vi "Add Page Attachements.vi"(6 "Parallel?":bool, 7 "Conf Printer in":refnum<class "VIDoc Printer - Confluence.lvclass">, 8 "error in (no error)":errorcluster, 9 "Msg Chain in":string, 10 "Attachments":set{path}(c389), 11 "Page in":refnum<class "Page.lvclass">) -> (0 "error out":errorcluster, 3 "Page out":refnum<class "Page.lvclass">, 5 "Conf Printer out":refnum<class "VIDoc Printer - Confluence.lvclass">)   [LabVIEW 2023, in "VIDoc Printer - Confluence.lvlib" / "VIDoc Printer - Confluence.lvclass"]
uses:
  VIDoc Printer - Confluence.lvclass
  C:/projects/DMC/GitHub/DMC CLI VIDoc/Source/Documentation Generation/Printers/Printer/VIDoc Printer.lvclass
  <userlib>/_PetranWay/LabVIEW Confluence API/Source/Confluence/Page/Page.lvclass
  <userlib>/_PetranWay/LabVIEW Confluence API/Source/Confluence/Page/Page.lvclass/Page.ctl
  <userlib>/_PetranWay/LabVIEW Confluence API/Source/Confluence/Page/Accessors/Read ID.vi
  VIDoc Printer - Confluence.lvclass/VIDoc Printer - Confluence.ctl
  Printer/VIDoc Printer.lvclass
  UI Interaction/UI Interaction.lvclass
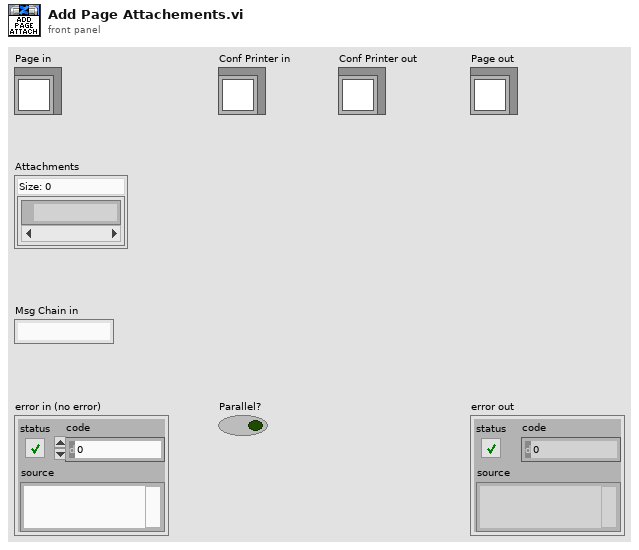
[diagram p1: front panel]
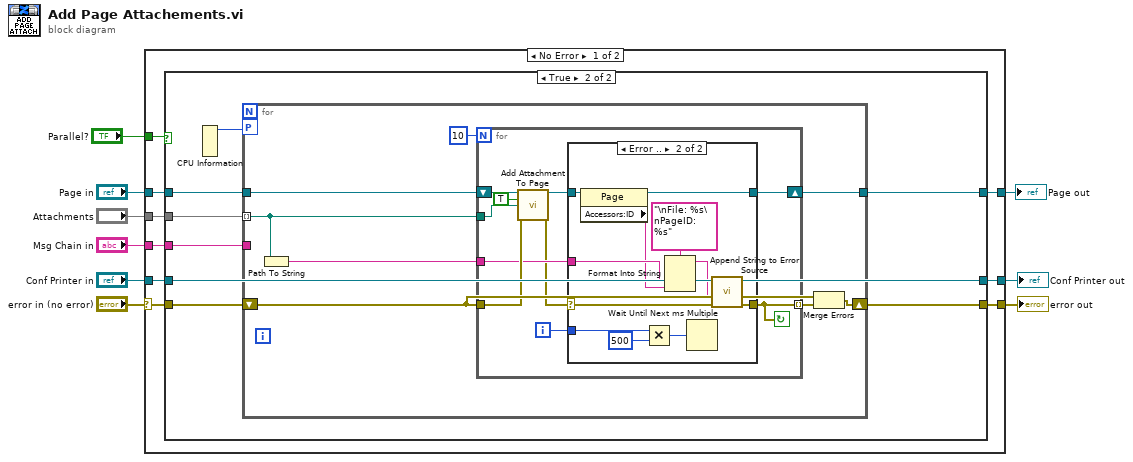
[diagram p0: block diagram]
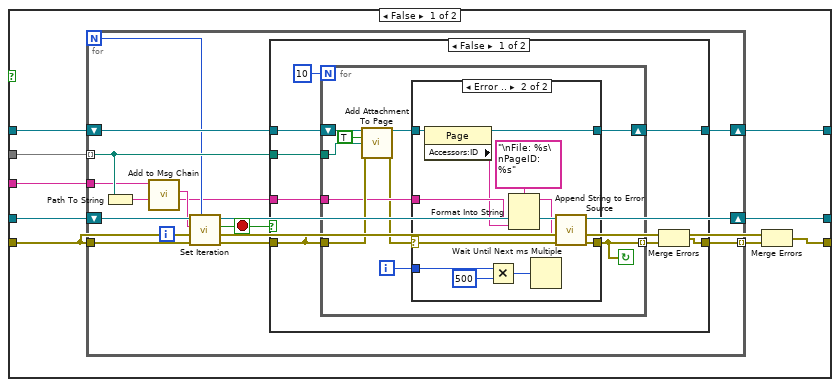
[diagram p2: hidden frame]
diagram:
  n1 = case shown="No Error" "error in (no error)" {
    selector: "error in (no error)" -> [w13 w116]
    tunnel: [w18 w115] -> w9
    tunnel: "Conf Printer in" -> [w17 w115]
    tunnel: "Attachments" -> [w16 _]
    tunnel: "Msg Chain in" -> [w15 _]
    tunnel: "Page in" -> [w14 w114]
    tunnel: [w12 w116] -> w3
    tunnel: [w11 w114] -> w2
    tunnel: "Parallel?" -> [w10 _]
    frame No Error {
      n2 = case shown="True" w10 {
        tunnel: [w27 w75] -> w18
        tunnel: w17 -> [w26 w75]
        tunnel: w16 -> [w25 w82]
        tunnel: w15 -> [w24 w81]
        tunnel: w14 -> [w23 w80]
        tunnel: w13 -> [w19 w79]
        tunnel: [w20 w78] -> w12
        tunnel: [w21 w77] -> w11
        frame False {
          n3 = for {
            N -> [w34]
            tunnel: w25 -> [w40] mode=indexing
            tunnel: w24 -> [w32]
            tunnel: w19 -> [w38]
            tunnel: [w39] -> w22 mode=indexing
            shift-right: [w35] -> w27
            shift-left: w26 -> [w36]
            shift-right: [w30] -> w21
            shift-left: w23 -> [w41]
            i -> [w33]
            stop <- w29 stop-if-true
            n4 = Path To String(path=w40) -> (string=w28:string)
            n5 = call "Add to Msg Chain.vi"("New"=w28, "Msg Chain in"=w32) -> ("Msg Chain out"=w31:string)  [unwired: 9 in]
            n6 = call "Set Iteration.vi"("Progress Max"=w34, "error in (no error)"=w38, "Progress Value"=w33, "Message (No Message Update)"=w31, "VIDoc Printer In"=w36) -> ("error out"=w37:errorcluster, "Abort?"=w29:bool, "VIDoc Printer Out"=w35:refnum<class "VIDoc Printer - Confluence.lvclass">)  [unwired: 4 in]
            n7 = case shown="False" w29 {
              tunnel: w41 -> [w49 w73]
              tunnel: w40 -> [w48 _]
              tunnel: [w43 w74] -> w39
              tunnel: w37 -> [w42 w74]
              tunnel: [w46 w73] -> w30
              tunnel: w28 -> [w44 _]
              frame False {
                n8 = for {
                  N: 10 -> [_]
                  tunnel: w48 -> [w58]
                  shift-right: [w55] -> w46
                  shift-left: w49 -> [w59]
                  tunnel: w42 -> [w57]
                  tunnel: [w56] -> w47 mode=indexing
                  tunnel: w44 -> [w53]
                  i -> [w52]
                  stop <- w56 continue-if-true
                  n9 = call-dynamic "Add Attachment To Page.vi"("Page"=w59, "Force Update / Upload"=TRUE, "File"=w58, "error in (no error)"=w57) -> ("Page"=w54:refnum<class "Page.lvclass">, "error out"=w50:errorcluster)  [unwired: 8 in, 2 out]
                  n10 = case shown="Error .." w50 {
                    selector: w50 -> [w61 w72]
                    tunnel: [w61 w71] -> w56
                    tunnel: [w60 w66] -> w55
                    tunnel: w54 -> [w60 w70]
                    tunnel: w53 -> [_ w67]
                    tunnel: w52 -> [_ w64]
                    frame No Error {
                    }
                    frame Error {
                      n11 = property class="Page"(reference=w70) -> (reference out=w66:refnum<class "Page.lvclass">, "Accessors:ID"=w65:string)  [unwired: 1 in, 1 out]
                      n12 = Multiply(x=w64, y=500) -> (x*y=w63:i32)
                      n13 = Format Into String(format string="\nFile: %s\nPageID: %s", w67, w65) -> (resulting string=w68:string)  [unwired: 2 in, 1 out]
                      n14 = Wait Until Next ms Multiple(millisecond multiple=w63) -> ()  [unwired: 1 out]
                      n15 = call "Append String to Error Source.vi"("Error In"=w72, "String to Append"=w68) -> ("Error Out"=w71:errorcluster)  [unwired: 9 in]
                    }
                  }
                }
                n16 = Merge Errors(w42, w47) -> (w43:errorcluster)
              }
              frame True {
              }
            }
          }
          n17 = Merge Errors(w19, w22) -> (w20:errorcluster)
        }
        frame True {
          n18 = CPU Information() -> (4:w76:i32)  [unwired: 3 out]
          n19 = for {
            tunnel: w82 -> [w89] mode=indexing
            tunnel: w81 -> [_]
            workers-P: w76 -> [_]
            shift-right: [w84] -> w78
            shift-left: w79 -> [w83]
            tunnel: w80 -> [w90]
            tunnel: [w87] -> w77
            n20 = Path To String(path=w89) -> (string=w86:string)
            n21 = for {
              N: 10 -> [_]
              tunnel: w89 -> [w99]
              shift-right: [w96] -> w87
              shift-left: w90 -> [w100]
              tunnel: w83 -> [w98]
              tunnel: [w97] -> w88 mode=indexing
              tunnel: w86 -> [w94]
              i -> [w93]
              stop <- w97 continue-if-true
              n22 = call-dynamic "Add Attachment To Page.vi"("Page"=w100, "Force Update / Upload"=TRUE, "File"=w99, "error in (no error)"=w98) -> ("Page"=w95:refnum<class "Page.lvclass">, "error out"=w91:errorcluster)  [unwired: 8 in, 2 out]
              n23 = case shown="Error .." w91 {
                selector: w91 -> [w102 w113]
                tunnel: [w102 w112] -> w97
                tunnel: [w101 w107] -> w96
                tunnel: w95 -> [w101 w111]
                tunnel: w94 -> [_ w108]
                tunnel: w93 -> [_ w105]
                frame No Error {
                }
                frame Error {
                  n24 = property class="Page"(reference=w111) -> (reference out=w107:refnum<class "Page.lvclass">, "Accessors:ID"=w106:string)  [unwired: 1 in, 1 out]
                  n25 = Multiply(x=w105, y=500) -> (x*y=w104:i32)
                  n26 = Format Into String(format string="\nFile: %s\nPageID: %s", w108, w106) -> (resulting string=w109:string)  [unwired: 2 in, 1 out]
                  n27 = Wait Until Next ms Multiple(millisecond multiple=w104) -> ()  [unwired: 1 out]
                  n28 = call "Append String to Error Source.vi"("Error In"=w113, "String to Append"=w109) -> ("Error Out"=w112:errorcluster)  [unwired: 9 in]
                }
              }
            }
            n29 = Merge Errors(w83, w88) -> (w84:errorcluster)
          }
        }
      }
    }
    frame Error {
    }
  }
  "Conf Printer out" <- w9
  "error out" <- w3
  "Page out" <- w2
